vi "is_path_invalid.vi"(1 "Path":path) -> (0 "Is invalid?":bool)   [LabVIEW 2015]
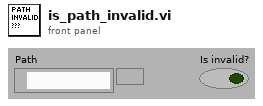
[diagram p1: front panel]
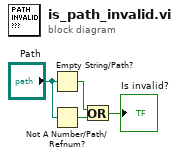
[diagram p0: block diagram]
diagram:
  n1 = Empty String/Path?(string/path="Path") -> (empty?=w1:bool)
  n2 = Not A Number/Path/Refnum?(number/path/refnum="Path") -> (NaN/Path/Refnum?=w3:bool)
  n3 = Or(x=w1, y=w3) -> (x .or. y?=→"Is invalid?":bool)
